vi "Obtain Request Events.vi"(8 "error in":errorcluster, 10 "Create New? (F)":bool) -> (0 "error out":errorcluster, 2 "Settings Request Events":T1)   [LabVIEW 2022 SP3, in "Settings.lvlib"]
doc: "This VI Obtains/Creates the Requests events that will be used for other modules to communicate with the module that owns this VI. These Requests events will be accessed only via Public API methods for this module.\n\n<b>NOTE</b>: The contents of this VI are automatically generated and modified by the <b>Tools > DQMH Consortium > DQMH</b> utilities. Consider using those utilities instead of making your own modifications to this VI.\n_____\nBased on DQMH Project Template 7.0.0.1280."
uses:
  Settings.lvlib
  Request Events--cluster.ctl
  Stop Argument--cluster.ctl
  Do Something Argument--cluster.ctl
  Do Something Else Argument--cluster.ctl
  Do Something Else and Wait for Reply Argument--cluster.ctl
  Do Something Else and Wait (Reply Payload)--cluster.ctl
  Show Panel Argument--cluster.ctl
  Hide Panel Argument--cluster.ctl
  Get Module Execution Status Argument--cluster.ctl
  Show Diagram Argument--cluster.ctl
  Prepare Argument--cluster.ctl
  Configure Argument--cluster.ctl
  Request UI Display Argument--cluster.ctl
  Framework/UI Manager/Module Display Scenarios.ctl
  Request UI Display (Reply Payload)--cluster.ctl
  Framework/UI Manager/UI Manager.lvlib
panel:
  # "NOTE: The contents of this VI are automatically generated and modified by the Tools > DQMH Consortium > DQMH utilities. Consider using those utilities instead of making your own modifications to this VI."
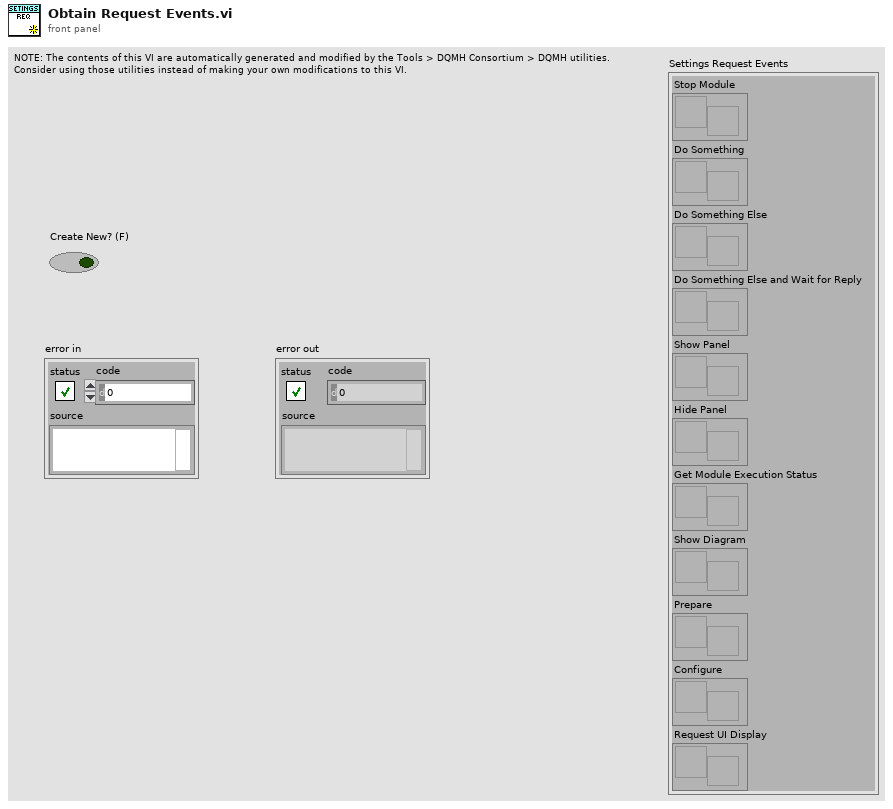
[diagram p1: front panel]
types:
  T1 = typedef "Settings.lvlib/Request Events--cluster.ctl" = cluster{"Stop Module":refnum<user-event>, "Do Something":refnum<user-event>, "Do Something Else":refnum<user-event>, "Do Something Else and Wait for Reply":refnum<user-event>, "Show Panel":refnum<user-event>, "Hide Panel":refnum<user-event>, "Get Module Execution Status":refnum<user-event>, "Show Diagram":refnum<user-event>, "Prepare":refnum<user-event>, "Configure":refnum<user-event>, "Request UI Display":refnum<user-event>}
  T2 = typedef "Settings.lvlib/Request UI Display Argument--cluster.ctl" = cluster{"Scenario":T3, "Wait Notifier":refnum<notifier>, "wait for reply":bool}
  T3 = typedef "UI Manager.lvlib/Module Display Scenarios.ctl" = enum16{"Stand-Alone", "Managed"}
  T4 = typedef "Settings.lvlib/Configure Argument--cluster.ctl" = cluster{"Boolean":bool}
  T5 = typedef "Settings.lvlib/Prepare Argument--cluster.ctl" = cluster{"Boolean":bool}
  T6 = typedef "Settings.lvlib/Hide Panel Argument--cluster.ctl" = cluster{"Hide Panel?":bool}
  T7 = typedef "Settings.lvlib/Show Panel Argument--cluster.ctl" = cluster{"Show Panel?":bool}
  T8 = typedef "Settings.lvlib/Show Diagram Argument--cluster.ctl" = cluster{"Debug?":bool}
  T9 = typedef "Settings.lvlib/Get Module Execution Status Argument--cluster.ctl" = cluster{"Running?":bool}
  T10 = typedef "Settings.lvlib/Do Something Else and Wait for Reply Argument--cluster.ctl" = cluster{"Do Something Else Msg":string, "X":dbl, "Wait Notifier":refnum<notifier>, "wait for reply":bool}
  T11 = typedef "Settings.lvlib/Do Something Else Argument--cluster.ctl" = cluster{"Do Something Else Msg":string, "X":dbl}
  T12 = typedef "Settings.lvlib/Do Something Argument--cluster.ctl" = cluster{"Do Something Msg":string}
  T13 = typedef "Settings.lvlib/Stop Argument--cluster.ctl" = cluster{"Origin":string, "Exit via Stop Module Req?":bool, "Wait for Module to stop?":bool}
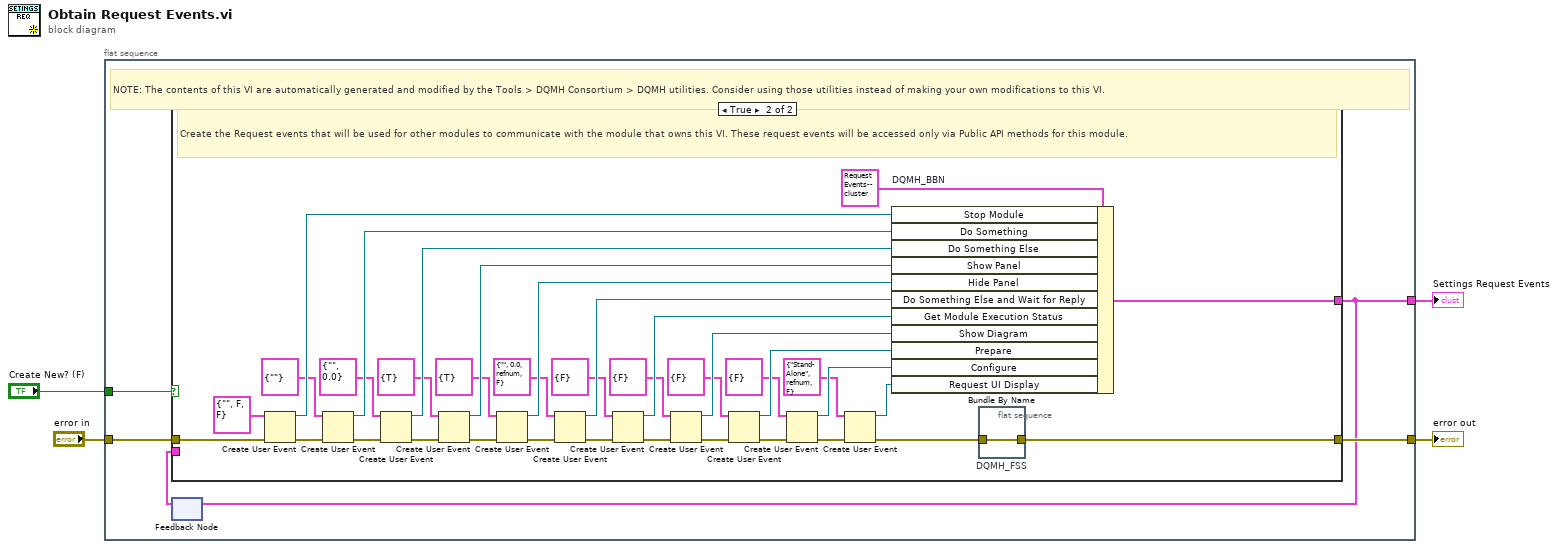
[diagram p0: block diagram]
diagram:
  n1 = flat-sequence {
    tunnel: [w9] -> w4
    tunnel: "error in" -> [w8]
    tunnel: [w6] -> w2
    tunnel: "Create New? (F)" -> [w5]
    frame #0 {
      # "NOTE: The contents of this VI are automatically generated and modified by the Tools > DQMH Consortium > DQMH utilities. Consider using those utilities instead of making your own modifications to this VI."
      n2 = feedback #1() -> (w7:T1)  [unwired: 1 in]
      n3 = case shown="True" w5 {
        tunnel: [w10 w29] -> w9
        tunnel: w8 -> [w10 w48]
        tunnel: [w11 w45] -> w6
        tunnel: w7 -> [w11 _]
        frame False {
          # "Obtain the Request events that were created in a previous call to this VI."
        }
        frame True {
          # "Create the Request events that will be used for other modules to communicate with the module that owns this VI. These request events will be accessed only via Public API methods for this module."
          n4 = Create User Event(user event datatype=T13 {"Origin"="", "Exit via Stop Module Req?"=FALSE, "Wait for Module to stop?"=FALSE} ("Stop Argument"), error in=w48) -> (user event=w46:refnum<user-event>, error out=w42:errorcluster)
          n5 = Create User Event(user event datatype=T12 {"Do Something Msg"=""} ("Do Something Argument"), error in=w42) -> (user event=w41:refnum<user-event>, error out=w40:errorcluster)
          n6 = Create User Event(user event datatype=T11 {"Do Something Else Msg"="", "X"=0.0} ("Do Something Else Argument"), error in=w40) -> (user event=w38:refnum<user-event>, error out=w37:errorcluster)
          n7 = Create User Event(user event datatype=T7 {"Show Panel?"=TRUE} ("Show Panel Argument"), error in=w37) -> (user event=w36:refnum<user-event>, error out=w35:errorcluster)
          n8 = Create User Event(user event datatype=T6 {"Hide Panel?"=TRUE} ("Hide Panel Argument"), error in=w35) -> (user event=w34:refnum<user-event>, error out=w33:errorcluster)
          n9 = Create User Event(user event datatype=T10 {"Do Something Else Msg"="", "X"=0.0, "Wait Notifier"=refnum, "wait for reply"=FALSE} ("Do Something Else and Wait for Reply Argument"), error in=w33) -> (user event=w32:refnum<user-event>, error out=w30:errorcluster)
          n10 = Create User Event(user event datatype=T9 {"Running?"=FALSE} ("Get Module Execution Status Argument"), error in=w30) -> (user event=w27:refnum<user-event>, error out=w28:errorcluster)
          n11 = Create User Event(user event datatype=T8 {"Debug?"=FALSE} ("Show Diagram Argument"), error in=w28) -> (user event=w24:refnum<user-event>, error out=w25:errorcluster)
          n12 = Create User Event(user event datatype=T5 {"Boolean"=FALSE} ("Prepare Argument"), error in=w25) -> (user event=w19:refnum<user-event>, error out=w20:errorcluster)
          n13 = Create User Event(user event datatype=T4 {"Boolean"=FALSE} ("Configure Argument"), error in=w20) -> (user event=w16:refnum<user-event>, error out=w17:errorcluster)
          n14 = Create User Event(user event datatype=T2 {"Scenario"=enum."Stand-Alone", "Wait Notifier"=refnum, "wait for reply"=FALSE} ("Request UI Display Argument"), error in=w17) -> (user event=w13:refnum<user-event>, error out=w14:errorcluster)
          n15 = Bundle By Name "DQMH_BBN"(cluster=T1 {"Stop Module"=refnum, "Do Something"=refnum, "Do Something Else"=refnum, "Do Something Else and Wait for Reply"=refnum, "Show Panel"=refnum, "Hide Panel"=refnum, "Get Module Execution Status"=refnum, "Show Diagram"=refnum, "Prepare"=refnum, "Configure"=refnum, "Request UI Display"=refnum} ("output cluster"), "Stop Module"=w46, "Do Something"=w41, "Do Something Else"=w38, "Show Panel"=w36, "Hide Panel"=w34, "Do Something Else and Wait for Reply"=w32, "Get Module Execution Status"=w27, "Show Diagram"=w24, "Prepare"=w19, "Configure"=w16, "Request UI Display"=w13) -> (w45:T1)
          n16 = flat-sequence "DQMH_FSS" {
            tunnel: w14 -> [w49]
            tunnel: [w49] -> w29
            frame #0 {
            }
          }
        }
      }
      n17 = feedback-in #1(w6) -> ()
    }
  }
  "Settings Request Events" <- w2
  "error out" <- w4
